vi "Compute Sample Length.vi"() -> (2 "Raw Smpl Len":i32)   [LabVIEW 2015, in "Tool Module.lvlib"]
uses:
  Tool Module.lvlib
  Tool Config/Tool Cfg.lvlib
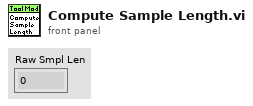
[diagram p1: front panel]
types:
  T1 = typedef "Tool Cfg.lvlib/_Tool Operation Config Cluster--typedef.ctl" = cluster{"Use Tool Cfg":bool, "Use Tool Cal":bool, "Fake Data?":bool, "Mode":i16, "Array Subset Length":i16, "nArrays to Read":i16, "Full Array Read Length":i16, "nSubarrays/Sensor":i16}
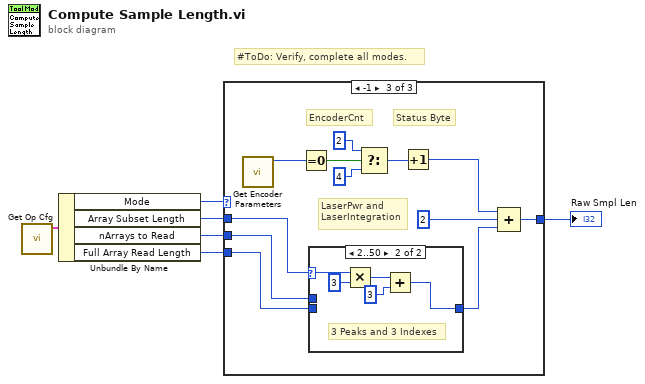
[diagram p0: block diagram]
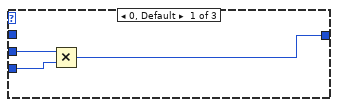
[diagram p2: hidden frame]
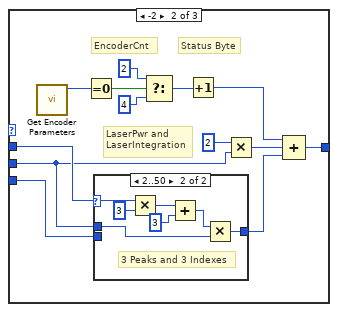
[diagram p3: hidden frame]
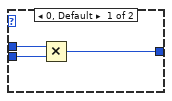
[diagram p4: hidden frame]
diagram:
  # "#ToDo: Verify, complete all modes."
  n1 = call "Get Op Cfg.vi"() -> ("Tool Operation Config"=w1:T1)  [unwired: 11 in]
  n2 = Unbundle By Name(w1) -> ("Mode"=w2:i16, "Array Subset Length"=w5:i16, "nArrays to Read"=w3:i16, "Full Array Read Length"=w4:i16)
  n3 = case shown="-1" w2 {
    tunnel: w3 -> [w9 w15 w38]
    tunnel: w4 -> [w8 w16 w39]
    tunnel: w5 -> [_ w17 w40]
    tunnel: [w7 w12 w36] -> w6
    frame 0, Default {
      n4 = Multiply(x=w9, y=w8) -> (x*y=w7:i16)
    }
    frame -2 {
      # "LaserPwr and\nLaserIntegration"
      # "Status Byte"
      # "EncoderCnt"
      n5 = call "Get Encoder Parameters.vi"() -> ("Encoder Size"=w10:u16)  [unwired: 9 in, 2 out]
      n6 = Equal To 0?(x=w10) -> (x = 0?=w22:bool)
      n7 = case shown="2..50" w17 {
        selector: w17 -> [_ w32]
        tunnel: w16 -> [w24 _]
        tunnel: w15 -> [w25 w27]
        tunnel: [w23 w26] -> w13
        frame 0, Default {
          n8 = Multiply(x=w25, y=w24) -> (x*y=w23:i16)
        }
        frame 2..50 {
          # "3 Peaks and 3 Indexes"
          n9 = Multiply(x=w32, y=i16 3) -> (x*y=w30:i16)
          n10 = Add(x=w30, y=i16 3) -> (x+y=w28:i16)
          n11 = Multiply(x=w28, y=w27) -> (x*y=w26:i16)
        }
      }
      n12 = Select(t=2 ("Raw Smpl Len"), s=w22, f=4 ("Raw Smpl Len")) -> (s? t:f=w19:i32)
      n13 = Increment(x=w19) -> (x+1=w11:i32)
      n14 = Multiply(x=2 ("Raw Smpl Len"), y=w15) -> (x*y=w14:i32)
      n15 = Compound Arithmetic op=ADD(w11, w14, w13) -> (w12:i32)
    }
    frame -1 {
      # "LaserPwr and\nLaserIntegration"
      # "Status Byte"
      # "EncoderCnt"
      n16 = call "Get Encoder Parameters.vi"() -> ("Encoder Size"=w33:u16)  [unwired: 9 in, 2 out]
      n17 = Equal To 0?(x=w33) -> (x = 0?=w44:bool)
      n18 = case shown="2..50" w40 {
        selector: w40 -> [_ w50]
        tunnel: w39 -> [w45 _]
        tunnel: w38 -> [_ _]
        tunnel: [w45 w46] -> w37
        frame 0, Default {
        }
        frame 2..50 {
          # "3 Peaks and 3 Indexes"
          n19 = Multiply(x=w50, y=i16 3) -> (x*y=w48:i16)
          n20 = Add(x=w48, y=i16 3) -> (x+y=w46:i16)
        }
      }
      n21 = Select(t=2 ("Raw Smpl Len"), s=w44, f=4 ("Raw Smpl Len")) -> (s? t:f=w41:i32)
      n22 = Increment(x=w41) -> (x+1=w35:i32)
      n23 = Compound Arithmetic op=ADD(w35, 2 ("Raw Smpl Len"), w37) -> (w36:i32)
    }
  }
  "Raw Smpl Len" <- w6
